vi "Init.vi"(8 "error in (no error)":errorcluster, 11 "DAQmx Delay Line in":refnum<class "DAQmx Delay Line.lvclass">) -> (0 "error out":errorcluster, 3 "DAQmx Delay Line out":refnum<class "DAQmx Delay Line.lvclass">)   [LabVIEW 2016, in "Delay Line.lvlib" / "DAQmx Delay Line.lvclass"]
uses:
  DAQmx Delay Line.lvclass
  Abstract Delay Line/Abstract Delay Line.lvclass
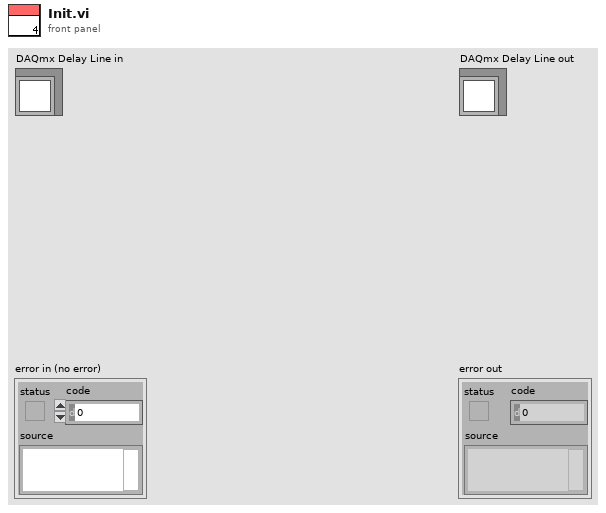
[diagram p1: front panel]
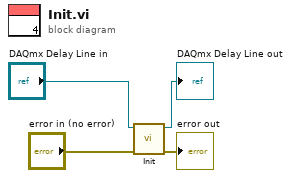
[diagram p0: block diagram]
diagram:
  n1 = call-parent "Init.vi"("error in (no error)"="error in (no error)", "Abstract Delay Line in"="DAQmx Delay Line in") -> ("error out"=→"error out":errorcluster, "Abstract Delay Line out"=→"DAQmx Delay Line out":refnum<class "DAQmx Delay Line.lvclass">)  [unwired: 8 in]
